vi "TeleopCommand.vi"(8 "error in (no error)":errorcluster, 10 "SubsystemData.lvclass":refnum<class "SubsystemData.lvclass">, 11 "Subsystem in":refnum<class "Subsystem.lvclass">) -> (0 "error out":errorcluster, 3 "Subsystem out":refnum<class "Subsystem.lvclass">)   [LabVIEW 2017, in "Subsystem.lvclass"]
uses:
  Subsystem.lvclass
  SubsystemData/SubsystemData.lvclass
  SubsystemData/CommandOrigin.ctl
  GetQueueRef.ctl
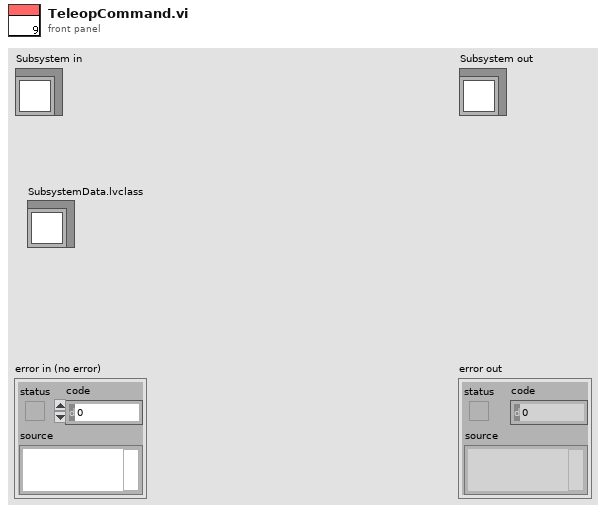
[diagram p1: front panel]
types:
  T1 = typedef "Subsystem.lvclass/GetQueueRef.ctl" = enum16{"Both", "Command", "Output"}
  T2 = typedef "SubsystemData.lvclass/CommandOrigin.ctl" = enum16{"Teleop", "Auto"}
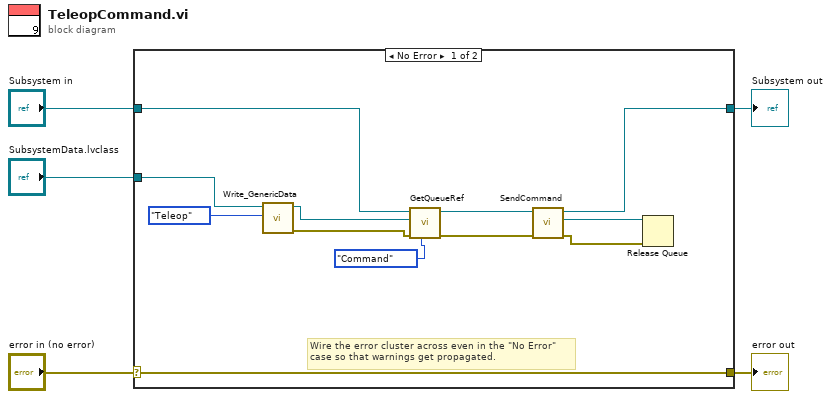
[diagram p0: block diagram]
diagram:
  n1 = case shown="No Error" "error in (no error)" {
    selector: "error in (no error)" -> [w17 w19]
    tunnel: [w17 w19] -> w4
    tunnel: [w7 w18] -> w2
    tunnel: "Subsystem in" -> [w10 w18]
    tunnel: "SubsystemData.lvclass" -> [w15 _]
    frame No Error {
      # "Wire the error cluster across even in the \"No Error\"\ncase so that warnings get propagated."
      n2 = call-dynamic "Write_GenericData.vi"("Data.CommandOrigin"=CommandOrigin."Teleop", "SubsystemData in"=w15) -> ("error out"=w8:errorcluster, "SubsystemData out"=w9:refnum<class "SubsystemData.lvclass">)  [unwired: 8 in]
      n3 = call-dynamic "GetQueueRef.vi"("GetQueueRef"=GetQueueRef."Command", "error in (no error)"=w8, "SubsystemData.lvclass"=w9, "Subsystem in"=w10) -> ("error out"=w12:errorcluster, "Subsystem out"=w11:refnum<class "Subsystem.lvclass">)  [unwired: 6 in]
      n4 = call-dynamic "SendCommand.vi"("error in (no error)"=w12, "Subsystem in"=w11) -> ("error out"=w13:errorcluster, "queue out"=w14:refnum<queue>, "Subsystem out"=w7:refnum<class "Subsystem.lvclass">)  [unwired: 7 in]
      n5 = Release Queue(queue=w14, error in (no error)=w13) -> ()  [unwired: 1 in, 3 out]
    }
    frame Error {
    }
  }
  "error out" <- w4
  "Subsystem out" <- w2
